vi "RSA306 hd2.vi"() -> ()   [LabVIEW 2016]
doc: "This VI demonstrates a simple procedure for setting up a spectrum analyzer, running an acquisition, and retrieving and plotting the waveform data.\n\nString indicators Binary WF Data and Sgl Float WF Data are initialized to empty strings. Waveform Graph is initialized to 0 for 100000 locations (just an arbitrary number for demonstration purposes).\n\ntkrsa6100 Initialize.vi opens the VISA Resource Name from the information entered by the user. It also presets the instrument by default to the Spectrum measurement. On completion it passes dup VISA Resource Name and error out to the following drivers.\n\nThe next VI to execute is tkrsa6100 Config Frequency.vi. Numeric control Center Freq (MHz)(50) is passed to the VI to set the center frequency to the default 50MHz value. The Set/Read Freq Setting (Set) is not wired since it defaults to SET, which is what is desired in this case. This is the case for all the configuration VI's in the example.\n\nThe next VI to execute is tkrsa6100 Config Spectrum Settings.vi. Enumerated control Spectrum Settings (CENTER FREQUENCY) is passed a Frequency Span constant and numeric control Freq Span (MHz) (40) to set the span to 40MHz.\n\nNext the reference level is set using tkrsa6100 Config RF Input.vi. Enumerated control Input Setting (REFERENCE LEVEL) is passed a Reference Level constant and numeric control Ref Level (dBm)(0) to set the reference level to 0dBm.\n\nNext the acquisition mode is set to single acquisition using tkrsa6100 Config Acquisition.vi. No parameters are passed since the default setting of this VI sets the acquisition mode to single.\n\nA single acquisition is then performed using tkrsa6100 Run Single Acquisition.vi. This VI sends an INIT command followed by a *OPC? Query. When the acquisition is completed the instrument returns a 1 and the next vi executes.\n\nThe binary waveform data is then retrieved by tkrsa6100 Spectrum Msmt Results.vi. The last acquisition data is retrieved by passing constant GET LAST ACQUISITION RESULT to enumerated input Run Acquisition and/or Get Result (RUN ACQUISITION & GET RESULT). The binary data is converted to a comma separated list of single precision floating point numbers by passing constant YES to enumerated input Convert Resp String (NO). The number of display points (total number of data bytes/4) is passed to a Spectral Display property node to scale the x axis of the graph. The binary data string from output Measurement Response String is copied to string indicator Binary WF Data. The converted binary data from output Converted Sgl Float Response String is copied to string indicator Sgl Float WF Data.\n\nSgl Float WF Data is then converted to an array by function Spreadsheet String to Array using a comma as the data separator. The output array is then passed to waveform graph Spectral Display for viewing.\n\nThe VISA Resource Name is closed using tkrsa6100 Close.vi."
panel:
  out "cursor diff":dbl
  out "# of Pts Between Cursors":dbl
  out "Cursor 1 X":dbl
  out "Cursor 0 X":dbl
  out "I & Q full":cluster{dbl[], "FFT {X}":dbl[]}[](graph)
  in  "stop":bool
  in  "FFT out From RSA":cluster{dbl[], "FFT {X}":dbl[]}(graph)={array[802 elements], "FFT {X}"=array[801 elements]}
  out "I & Q  partial":cluster{dbl[], dbl[]}[](graph)
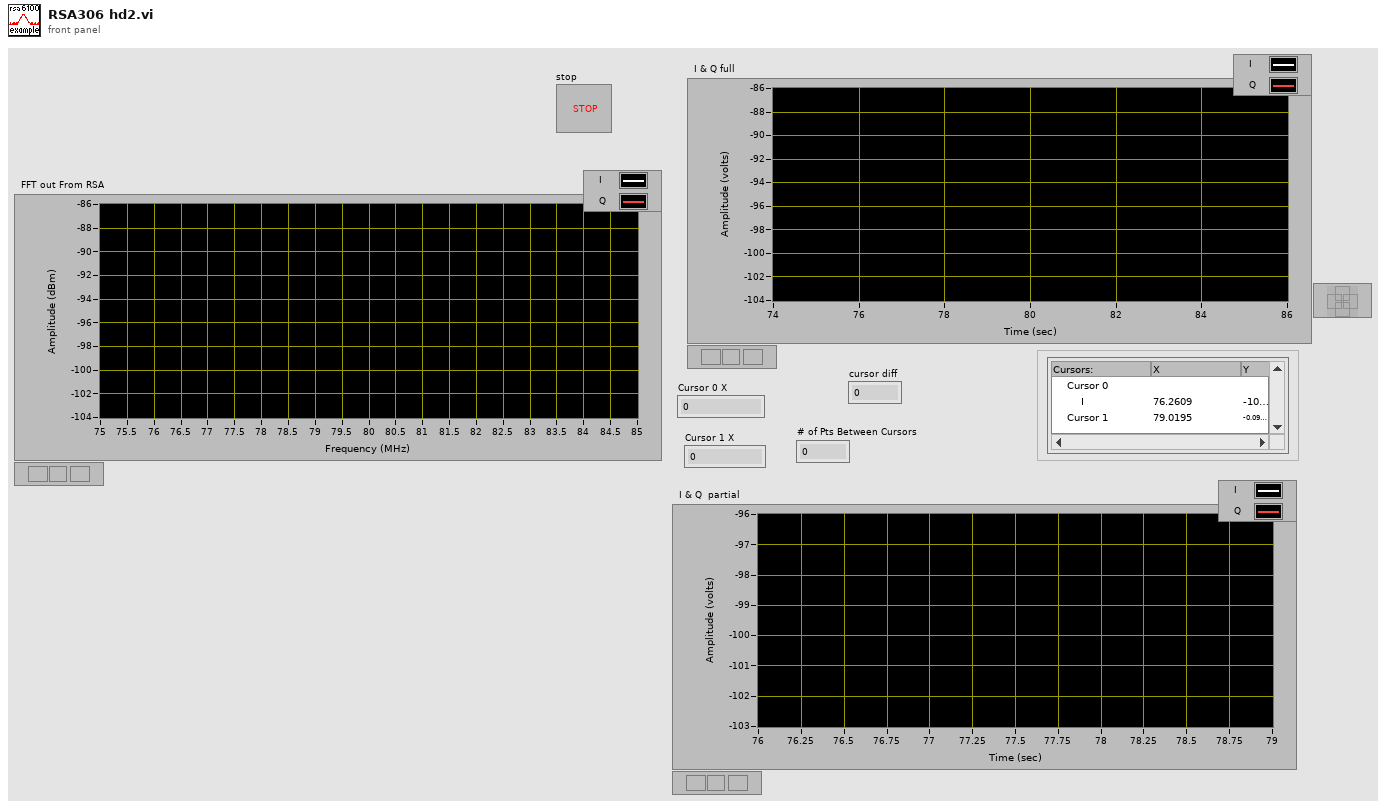
[diagram p1: front panel]
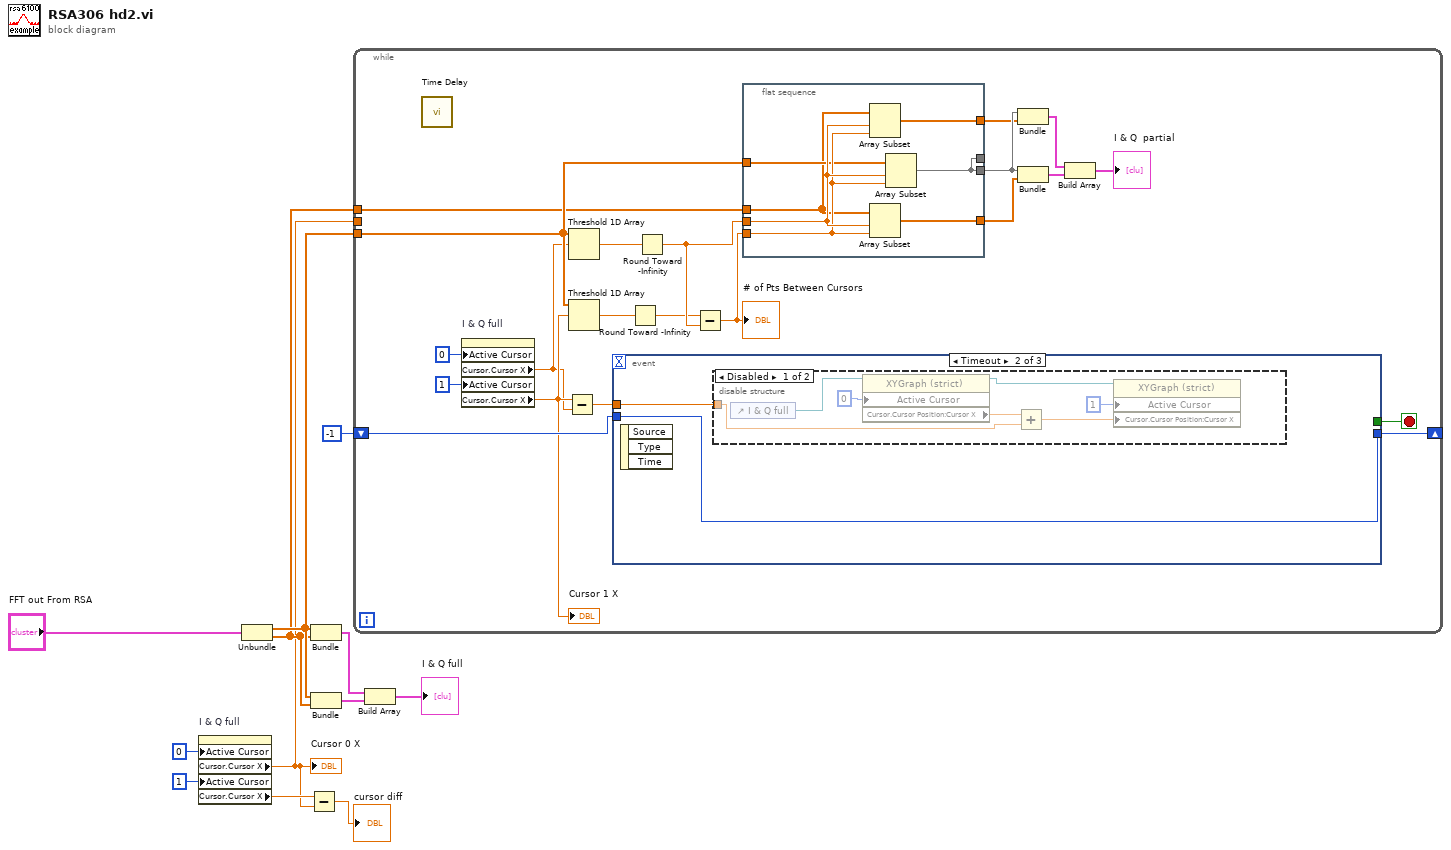
[diagram p0: block diagram]
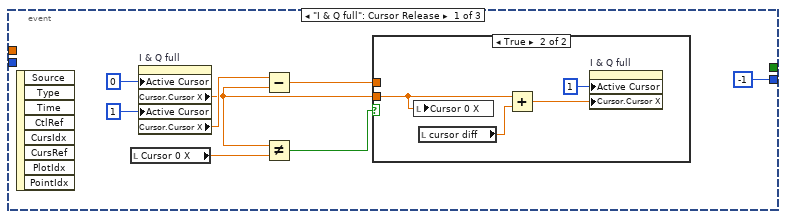
[diagram p2: hidden frame]
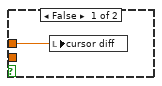
[diagram p3: hidden frame]
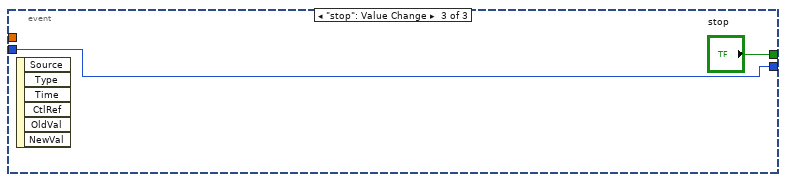
[diagram p5: hidden frame]
diagram:
  n1 = property on="I & Q full" class="XYGraph (strict)"("Active Cursor"=u32 0, "Active Cursor"=u32 1) -> ("Cursor.Cursor X"=w3:dbl, "Cursor.Cursor X"=w5:dbl)  [unwired: 2 in, 2 out]
  "Cursor 0 X" <- w3
  n2 = Unbundle("FFT out From RSA") -> (w8:dbl[], "FFT {X}"=w7:dbl[])
  n3 = Subtract(x=w5, y=w3) -> (x-y=→"cursor diff":dbl)
  n4 = Bundle(w8, "FFT {X}"=w7) -> (w11:cluster{dbl[], "FFT {X}":dbl[]})  [unwired: 1 in]
  n5 = Bundle(w8, "FFT {X}"=w7) -> (w12:cluster{dbl[], "FFT {X}":dbl[]})  [unwired: 1 in]
  n6 = while {
    tunnel: w8 -> [w25]
    shift-right: [w21] -> _
    shift-left: -1 -> [w22]
    tunnel: w7 -> [w16]
    tunnel: w3 -> [_]
    stop <- w20 stop-if-true
    n7 = call "Time Delay"() -> ()  [unwired: 11 in, 1 out]
    n8 = property on="I & Q full" class="XYGraph (strict)"("Active Cursor"=u32 0, "Active Cursor"=u32 1) -> ("Cursor.Cursor X"=w18:dbl, "Cursor.Cursor X"=w19:dbl)  [unwired: 2 in, 2 out]
    "Cursor 1 X" <- w19
    n9 = Subtract(x=w19, y=w18) -> (x-y=w17:dbl)
    n10 = Threshold 1D Array(2:w18, 3:w25) -> (0:w29:dbl)  [unwired: 1 in]
    n11 = Threshold 1D Array(2:w19, 3:w25) -> (0:w28:dbl)  [unwired: 1 in]
    n12 = event shown="[1] Timeout" {
      selector: _ -> [_ _ _]
      dyn-events: _ -> [_ _ _]
      timeout: _ -> [_ _ _]
      tunnel: [_ _ "stop"] -> w20
      tunnel: [-1 w48 w57] -> w21
      tunnel: w22 -> [_ w48 w57]
      tunnel: w17 -> [_ w47 _]
      event "I & Q full": Cursor Release {
        n13 = event-data() -> ()  [unwired: 1 in, 8 out]
        n14 = local read "Cursor 0 X"() -> (w38:dbl)
        n15 = property on="I & Q full" class="XYGraph (strict)"("Active Cursor"=u32 0, "Active Cursor"=u32 1) -> ("Cursor.Cursor X"=w35:dbl, "Cursor.Cursor X"=w36:dbl)  [unwired: 2 in, 2 out]
        n16 = Subtract(x=w36, y=w35) -> (x-y=w34:dbl)
        n17 = Not Equal?(x=w35, y=w38) -> (x != y?=w37:bool)
        n18 = case shown="True" w37 {
          tunnel: w35 -> [_ w43]
          tunnel: w34 -> [w42 _]
          frame False {
            n19 = local write "cursor diff"(w42) -> ()
          }
          frame True {
            n20 = local write "Cursor 0 X"(w43) -> ()
            n21 = local read "cursor diff"() -> (w45:dbl)
            n22 = Add(x=w43, y=w45) -> (x+y=w44:dbl)
            n23 = property on="I & Q full" class="XYGraph (strict)"("Active Cursor"=u32 1, "Cursor.Cursor X"=w44) -> ()  [unwired: 2 in, 2 out]
          }
        }
      }
      event Timeout {
        n24 = event-data() -> ()  [unwired: 1 in, 3 out]
        n25 = disable-structure shown="Disabled" {
          disable-tunnel: w47 -> [w49 _]
          frame Disabled {
            n26 = control-ref of="I & Q full"() -> (w50:refnum<vi>)
            n27 = property class="XYGraph (strict)"(reference=w50, "Active Cursor"=u32 0) -> (reference out=w53:refnum<vi>, "Cursor.Cursor Position:Cursor X"=w52:dbl)  [unwired: 1 in, 1 out]
            n28 = Add(x=w52, y=w49) -> (x+y=w51:dbl)
            n29 = property class="XYGraph (strict)"(reference=w53, "Active Cursor"=u32 1, "Cursor.Cursor Position:Cursor X"=w51) -> ()  [unwired: 1 in, 2 out]
          }
          frame Enabled {
          }
        }
      }
      event "stop": Value Change {
        n30 = event-data() -> ()  [unwired: 1 in, 6 out]
      }
    }
    n31 = Round Toward -Infinity(1:w28) -> (0:w26:dbl)
    n32 = Round Toward -Infinity(1:w29) -> (0:w27:dbl)
    n33 = Subtract(x=w26, y=w27) -> (x-y=w23:dbl)
    "# of Pts Between Cursors" <- w23
    n34 = flat-sequence {
      tunnel: [w64] -> w15
      tunnel: [w63] -> w14
      tunnel: w27 -> [w62]
      tunnel: w23 -> [w61]
      tunnel: w25 -> [w60]
      tunnel: [w59] -> _
      tunnel: [w59] -> w24
      tunnel: w16 -> [w58]
      frame #0 {
        n35 = Array Subset(array=w58, index=w62, length=w61) -> (w64:dbl[])
        n36 = Array Subset(array=w58, index=w62, length=w61) -> (w63:dbl[])
        n37 = Array Subset(array=w60, index=w62, length=w61) -> (w59:dbl[])
      }
    }
    n38 = Bundle(w24, w15) -> (w32:cluster{dbl[], dbl[]})  [unwired: 1 in]
    n39 = Bundle(w24, w14) -> (w33:cluster{dbl[], dbl[]})  [unwired: 1 in]
    n40 = Build Array(w32, w33) -> (→"I & Q  partial":cluster{dbl[], dbl[]}[])
  }
  n41 = Build Array(w11, w12) -> (→"I & Q full":cluster{dbl[], "FFT {X}":dbl[]}[])
